vi "LACallback.vi"(8 "Error In":errorcluster, 10 "ToolReturn":cluster{"id":string, "result":variant}, 11 "LiteAgent In":T1) -> (0 "Error Out":errorcluster, 3 "LiteAgent Out":T1)   [LabVIEW 2017, in "LiteAgentSDK.lvlib"]
uses:
  LiteAgentSDK.lvlib
  C:/Users/Jan/Projects/LiteAgentSDK-LabVIEW/Source/Bin/LiteAgentSDK.LabVIEW.dll
  Bin/LiteAgentSDK.LabVIEW.dll
  <vilib>/LVH/i3 JSON/i3-json.lvlib
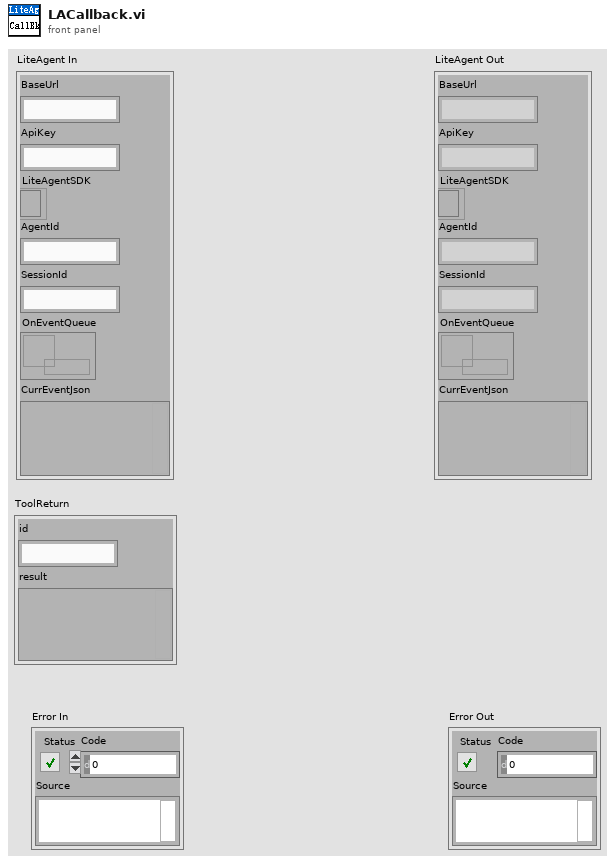
[diagram p1: front panel]
types:
  T1 = cluster{"BaseUrl":string, "ApiKey":string, "LiteAgentSDK":refnum<k24>, "AgentId":string, "SessionId":string, "OnEventQueue":refnum<queue>, "CurrEventJson":variant}
  T2 = cluster{"functionCallId":string, "result":string}
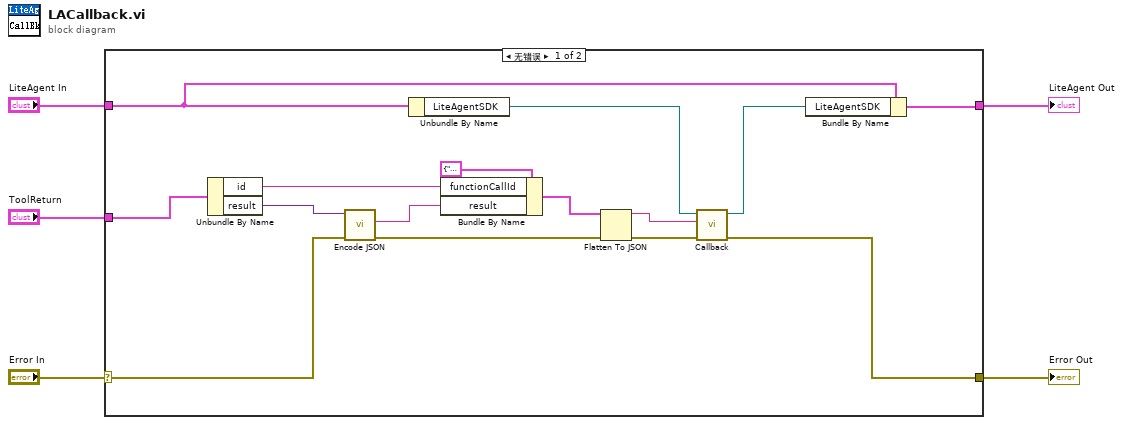
[diagram p0: block diagram]
diagram:
  n1 = case shown="无错误" "Error In" {
    selector: "Error In" -> [w13 w22]
    tunnel: [w18 w22] -> w4
    tunnel: "LiteAgent In" -> [w20 w21]
    tunnel: [w19 w21] -> w2
    tunnel: "ToolReturn" -> [w14 _]
    frame No Error {
      n2 = Unbundle By Name(w14) -> ("id"=w11:string, "result"=w12:variant)
      n3 = call <vilib>:"Encode JSON.vi"("error in (no error)"=w13, "JSON Tree"=w12) -> ("error out"=w8:errorcluster, "String"=w10:string)  [unwired: 4 in]
      n4 = Unbundle By Name(w20) -> ("LiteAgentSDK"=w17:refnum<k24>)
      n5 = Bundle By Name(cluster=T2 {"functionCallId"="", "result"=""}, "functionCallId"=w11, "result"=w10) -> (w9:T2)
      n6 = Flatten To JSON(anything=w9, error in (no error)=w8) -> (JSON string=w6:string, 11:w7:errorcluster)  [unwired: 1 in]
      n7 = call "Callback.vi"("Error Input"=w7, "ToolReturnJson"=w6, "LiteAgentSDK Input"=w17) -> ("Error Output"=w18:errorcluster, "LiteAgentSDK Output"=w16:refnum<k24>)  [unwired: 7 in]
      n8 = Bundle By Name(cluster=w20, "LiteAgentSDK"=w16) -> (w19:T1)
    }
    frame Error {
    }
  }
  "Error Out" <- w4
  "LiteAgent Out" <- w2
